vi "Save.vi"(8 "error in":errorcluster, 10 "file path":path, 11 "SequenceRepo in":refnum<class "SequenceRepo.lvclass">) -> (0 "error out":errorcluster, 3 "SequenceRepo out":refnum<class "SequenceRepo.lvclass">)   [LabVIEW 2015, in "SequenceRepo.lvclass"]
doc: "Calls the Read Tree VI to have an updated version of the Repo and then saves the repo information into the XML file.Copyright 2017 National Instruments Corporation\n\nLicensed under the Apache License, Version 2.0 (the \"License\"); you may not use this file except in compliance with the License. You may obtain a copy of the License at http://www.apache.org/licenses/LICENSE-2.0\nUnless required by applicable law or agreed to in writing, software distributed under the License is distributed on an \"AS IS\" BASIS, WITHOUT WARRANTIES OR CONDITIONS OF ANY KIND, either express or implied. See the License for the specific language governing permissions and limitations under the License."
uses:
  SequenceRepo.lvclass
  SequenceRepo.lvclass/SequenceRepo.ctl
  <vilib>/Utility/file.llb/Write Delimited Spreadsheet (string).vi
  Prototype/classes/Sequence/Config/Sequence Config.lvclass
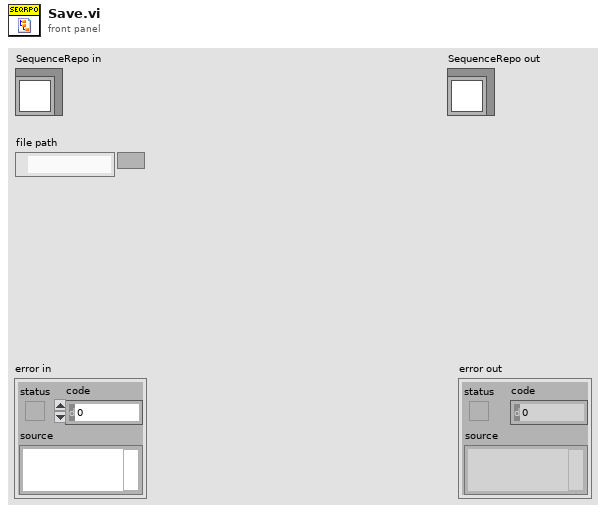
[diagram p1: front panel]
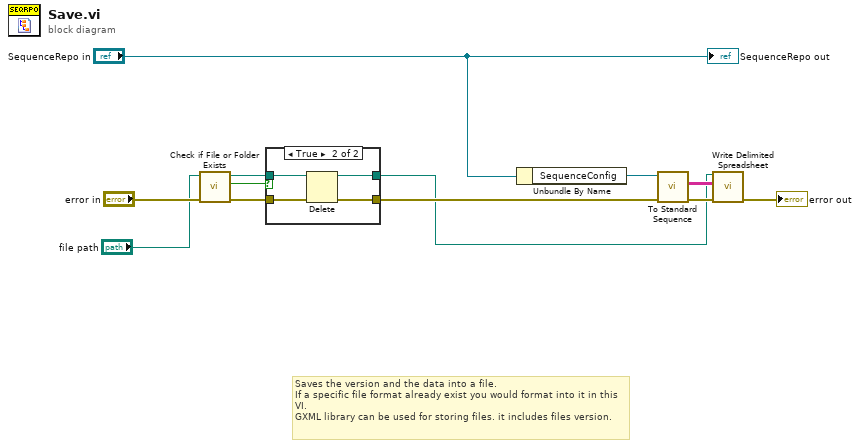
[diagram p0: block diagram]
diagram:
  # "Saves the version and the data into a file.\nIf a specific file format already exist you would format into it in this VI.\nGXML library can be used for storing files. it includes files version."
  n1 = call <vilib>:"Check if File or Folder Exists.vi"("error in (no error)"="error in", "path"="file path") -> ("error out"=w5:errorcluster, "file or folder exists?"=w7:bool, "dup path"=w6:path)  [unwired: 7 in]
  n2 = case shown="True" w7 {
    tunnel: w6 -> [w14 w18]
    tunnel: [w14 w17] -> w1
    tunnel: w5 -> [w13 w16]
    tunnel: [w13 w15] -> w3
    frame False {
    }
    frame True {
      n3 = Delete(path (use dialog)=w18, error in=w16) -> (deleted path=w17:path, error out=w15:errorcluster)  [unwired: 3 in, 1 out]
    }
  }
  n4 = Unbundle By Name("SequenceRepo in") -> ("SequenceConfig"=w11:refnum<class "Sequence Config.lvclass">)
  n5 = call-dynamic "To Standard Sequence.vi"("error in (no error)"=w3, "Sequence Config in"=w11) -> ("error out"=w10:errorcluster, "Standard Sequence"=w8:string[][])  [unwired: 7 in, 1 out]
  n6 = call-poly <vilib>:"Write Delimited Spreadsheet.vi"("file path (dialog if empty)"=w1, "2D data"=w8, "error in (no error)"=w10) -> ("error out"=→"error out":errorcluster)  [unwired: 11 in, 1 out]
  "SequenceRepo out" <- "SequenceRepo in"
